vi "Read Test Data.vi"(11 "Message Test":refnum<class "TestManagerMsg.Test.lvclass">) -> (2 "Test Data":T1, 3 "Message Test out":refnum<class "TestManagerMsg.Test.lvclass">)   [LabVIEW 2013, in "Caraya.lvlib" / "TestManagerMsg.Test.lvclass"]
uses:
  TestManagerMsg.Test.lvclass
  Test-Data -- cluster.ctl
  TestManagerMsg.Test.lvclass/TestManagerMsg.Test.ctl
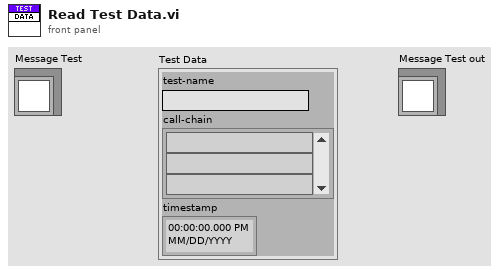
[diagram p1: front panel]
types:
  T1 = typedef "Caraya.lvlib/TestManagerMsg.Test.lvclass/Test-Data -- cluster.ctl" = cluster{"test-name":string, "call-chain":string[], "timestamp":timestamp}
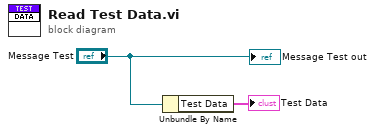
[diagram p0: block diagram]
diagram:
  n1 = Unbundle By Name("Message Test") -> ("Test Data"=→"Test Data":T1)
  "Message Test out" <- "Message Test"
